vi "Execute.vi"(8 "error in (no error)":errorcluster, 10 "Abstract Consumer in":refnum<class "Abstract Consumer.lvclass">, 11 "Switch Disconnect All Message in":refnum<class "Switch Disconnect All Message.lvclass">) -> (0 "error out":errorcluster, 1 "Abstract Response out":refnum<class "Abstract Response Message.lvclass">, 2 "Abstract Consumer out":refnum<class "Abstract Consumer.lvclass">, 3 "Switch Disconnect All Message out":refnum<class "Switch Disconnect All Message.lvclass">, 4 "Stop?":bool)   [LabVIEW 2017, in "Messaging.lvlib" / "Switch Disconnect All Message.lvclass"]
uses:
  Switch Disconnect All Message.lvclass
  Consumer/Abstract Consumer/Abstract Consumer.lvclass
  Message/Abstract Response Message/Abstract Response Message.lvclass
  Abstract Switch Consumer/Abstract Switch Consumer.lvclass
  C:/github/niveristand-custom-device-message-library/Source/Consumer/Abstract Consumer/Abstract Consumer.lvclass
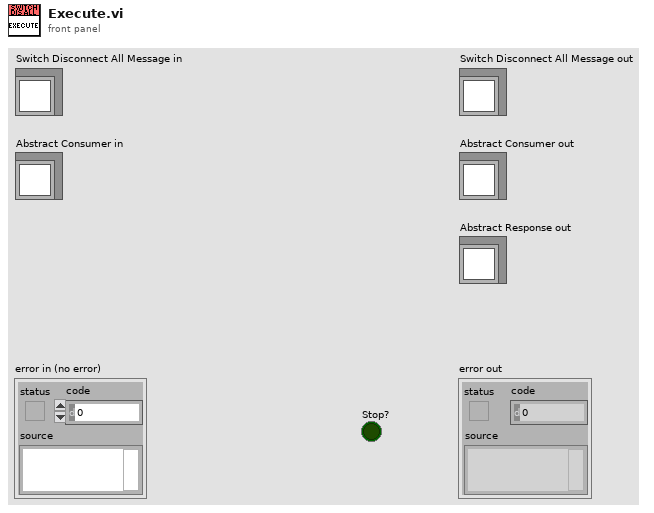
[diagram p1: front panel]
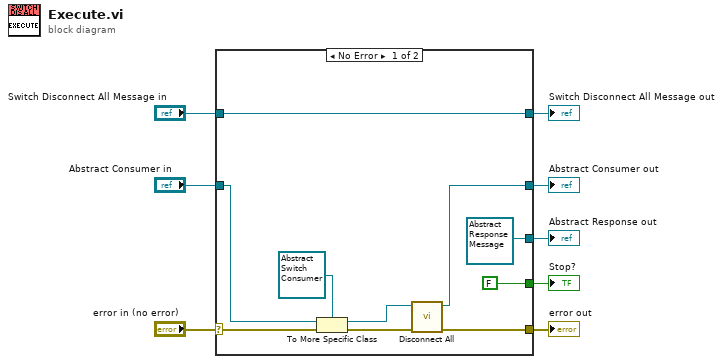
[diagram p0: block diagram]
diagram:
  n1 = case shown="No Error" "error in (no error)" {
    selector: "error in (no error)" -> [w14 w21]
    tunnel: [w12 w21] -> w7
    tunnel: [w17 w20] -> w6
    tunnel: "Switch Disconnect All Message in" -> [w17 w20]
    tunnel: [w10 w19] -> w4
    tunnel: "Abstract Consumer in" -> [w16 w19]
    tunnel: [FALSE ("Stop?") _] -> w2
    tunnel: [refnum<class "Abstract Response Message.lvclass"> refnum ("Abstract Response out") _] -> w1
    frame No Error {
      n2 = To More Specific Class(target class=refnum<class "Abstract Switch Consumer.lvclass"> refnum ("Message Queue Library.lvlib:Abstract Switch Consumer.lvclass"), reference=w16, error in=w14) -> (specific class reference=w11:refnum<class "Abstract Switch Consumer.lvclass">, error out=w13:errorcluster)
      n3 = call-dynamic "Disconnect All.vi"("error in (no error)"=w13, "Abstract Switch Consumer in"=w11) -> ("error out"=w12:errorcluster, "Abstract Switch Consumer out"=w10:refnum<class "Abstract Switch Consumer.lvclass">)  [unwired: 8 in]
    }
    frame Error {
    }
  }
  "error out" <- w7
  "Switch Disconnect All Message out" <- w6
  "Abstract Consumer out" <- w4
  "Stop?" <- w2
  "Abstract Response out" <- w1
